vi "Open VI.vi"(8 "error in":errorcluster, 11 "vi path":path=path "C:/Users/lubo/Documents/LabView/LabVIEW-Universal-Transcriptor/Test/Example Test 1.vi") -> (0 "error out":errorcluster, 3 "vi reference":refnum<vi>)   [LabVIEW 2014]
doc: "Open VI specified by absolute path."
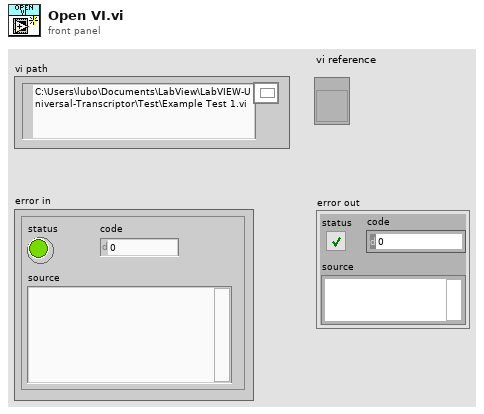
[diagram p1: front panel]
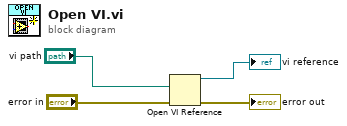
[diagram p0: block diagram]
diagram:
  n1 = Open VI Reference(vi path="vi path", error in (no error)="error in") -> (vi reference=→"vi reference":refnum<vi>, error out=→"error out":errorcluster)  [unwired: 4 in]
